vi "Facade.vi"(0 "Data In":T9, 2 "Display State In":T5, 3 "Container State":T8) -> (6 "Data Out":T9, 7 "Display State Out":T5, 8 "Action":T4)   [LabVIEW 2020, in "PXISlotGP.xctl"]
uses:
  PXISlotGP.xctl
  Data.ctl
  <vilib>/_xctls/Container State.ctl
  State.ctl
  PXISlot XControl/Connector Type.ctl
  AOAIRefs.ctl
  <vilib>/_xctls/Action.ctl
  <vilib>/_xctls/XControlSupport.lvlib
panel:
  in  "Tab panel":T1(tab) caption="SLOT X"
  in  "None":cluster{"String":string}
  in  "PXI-4461":T2 caption="Slot X"
  in  "BNC-2110":T3 caption="Slot X"
  in  "BNC-2090":T3 caption="Slot X"
types:
  T1 = enum32{"None", "PXI-4461", "BNC-2110", "BNC-2090"}
  T2 = cluster{"AI0":u16, "AI1":u16, "AO0":u16, "AO1":u16}
  T3 = cluster{"AI0":u16, "AI1":u16, "AI2":u16, "AI3":u16, "AI4":u16, "AI5":u16, "AI6":u16, "AI7":u16, "AO0":u16, "AO1":u16, "Trigger":string}
  T4 = typedef "XControlSupport.lvlib/Action.ctl" = cluster{"Data Changed?":bool, "State Changed?":bool, "Action Name":string}
  T5 = typedef "PXISlotGP.xctl/State.ctl" = cluster{"Connector Type":T6, "Hide unused":bool, "Trigger Visible":bool, "TabRef":refnum<vi>, "ConnRefs":refnum<vi>[], "PaneRef":refnum<vi>, "AOAIRefs":T7[], "TriggerRefs":refnum<vi>[], "check data":bool, "Name":string, "Events":cluster{"Type changed":refnum<user-event>}}
  T6 = typedef "Connector Type.ctl" = enum16{"None", "PXI-4461", "BNC-2110", "BNC-2090", "PXIe-4463", "PXIe-4464"}
  T7 = typedef "AOAIRefs.ctl" = cluster{"AORefs":refnum<vi>[], "AIRefs":refnum<vi>[]}
  T8 = typedef "XControlSupport.lvlib/Container State.ctl" = cluster{"Indicator?":bool, "Run Mode?":bool, " Refnum":refnum<vi>}
  T9 = typedef "PXISlotGP.xctl/Data.ctl" = cluster{"Outputs":string[], "Inputs":string[]}
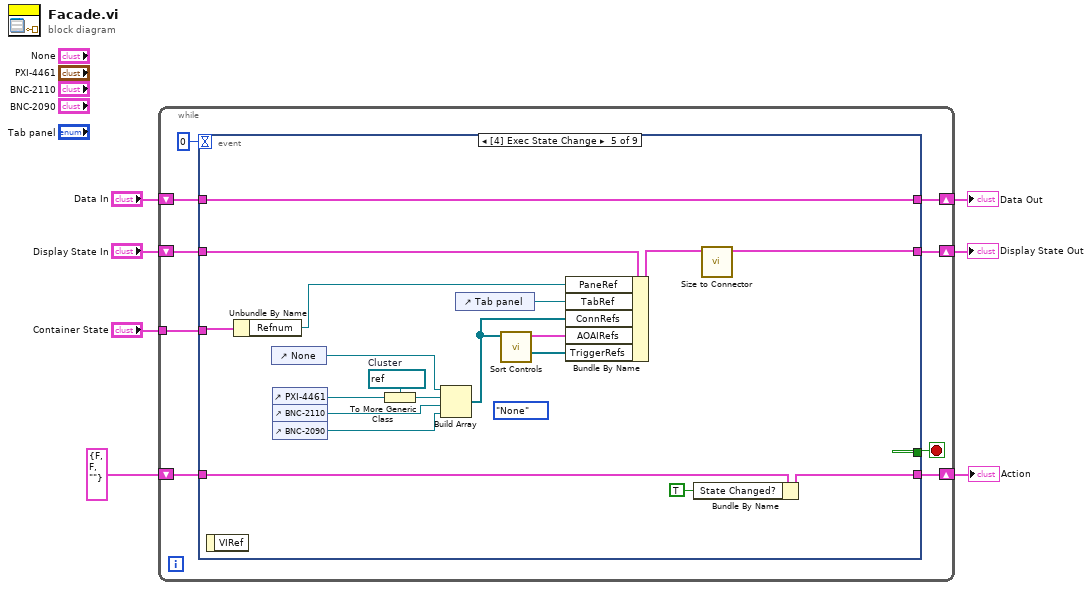
[diagram p0: block diagram]
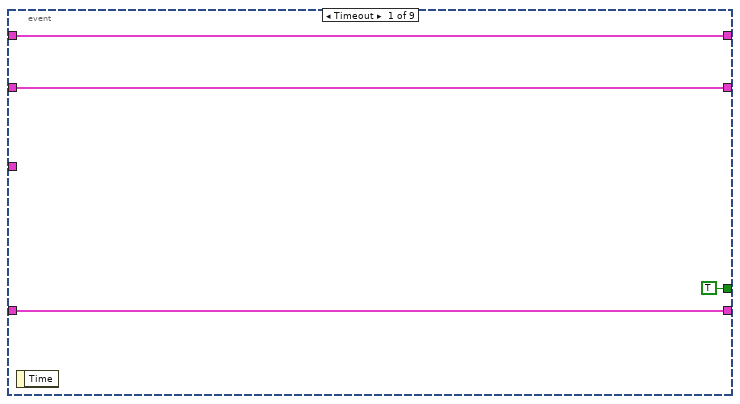
[diagram p2: hidden frame]
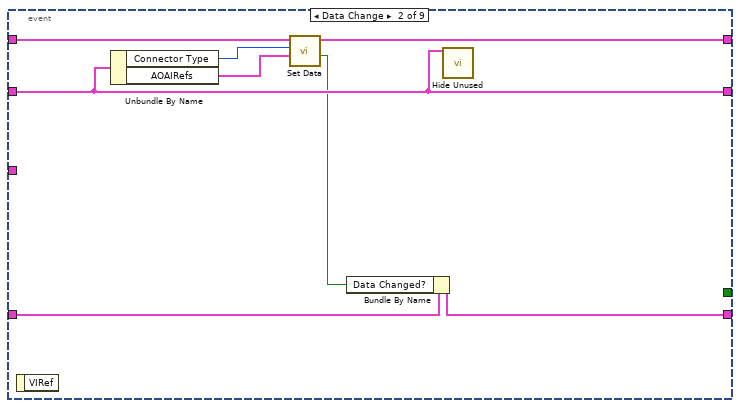
[diagram p3: hidden frame]
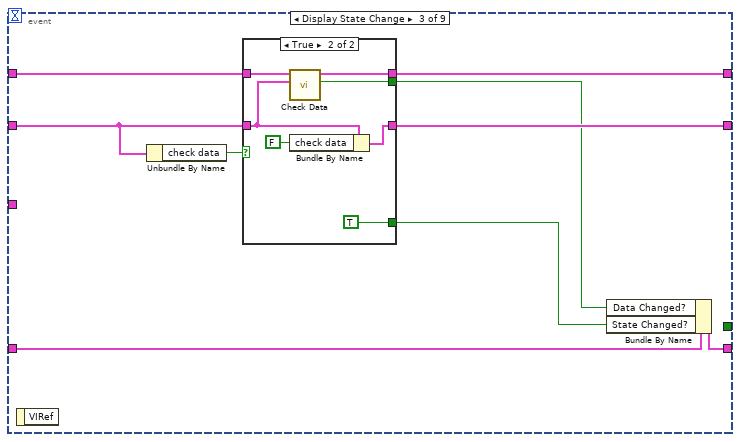
[diagram p4: hidden frame]
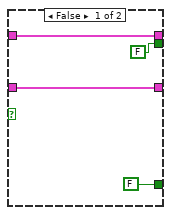
[diagram p5: hidden frame]
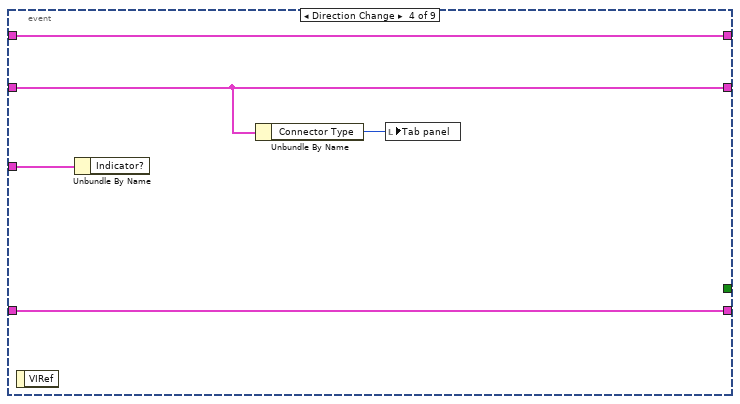
[diagram p6: hidden frame]
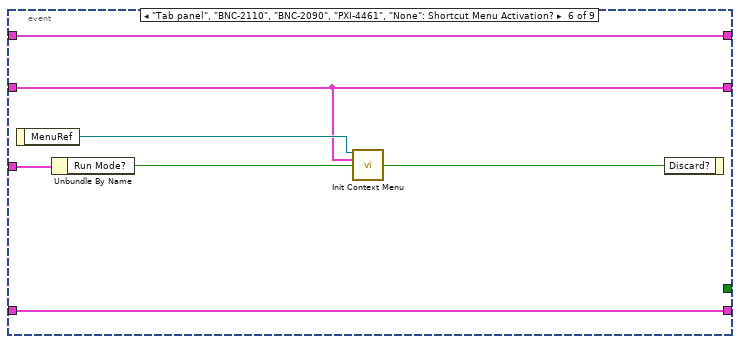
[diagram p7: hidden frame]
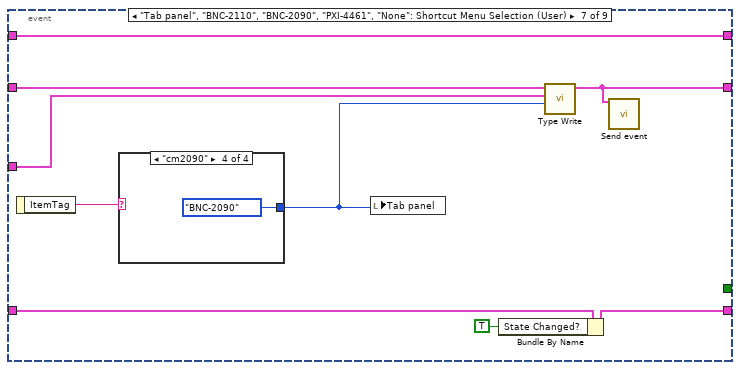
[diagram p8: hidden frame]
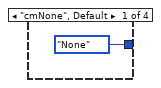
[diagram p9: hidden frame]
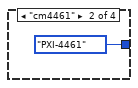
[diagram p10: hidden frame]
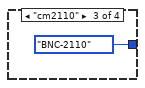
[diagram p11: hidden frame]
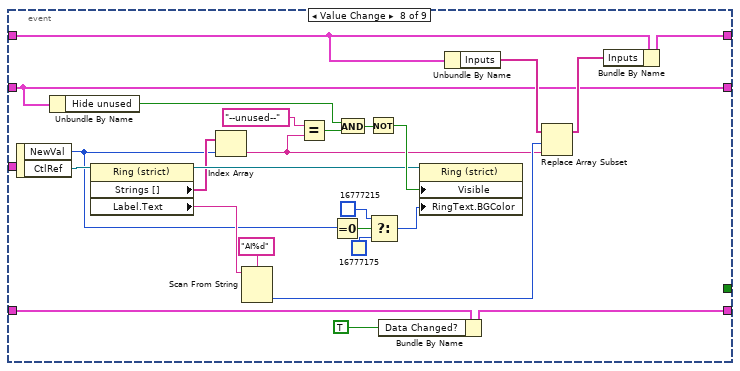
[diagram p12: hidden frame]
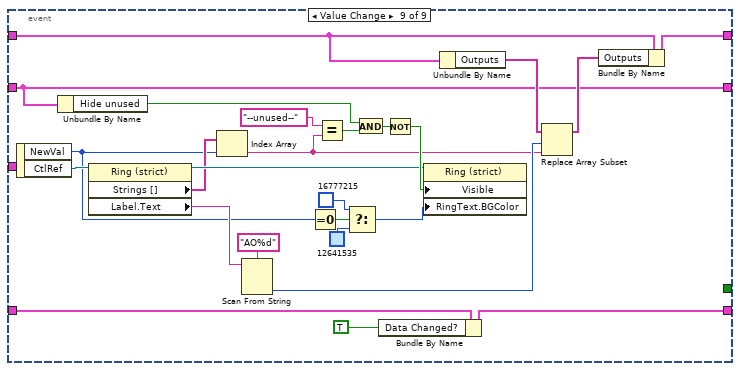
[diagram p13: hidden frame]
diagram:
  n1 = while {
    shift-right: [w15] -> w4
    shift-left: "Display State In" -> [w16]
    tunnel: "Container State" -> [w12]
    shift-right: [w10] -> w7
    shift-left: "Data In" -> [w11]
    shift-right: [w8] -> w2
    shift-left: T4 {"Data Changed?"=FALSE, "State Changed?"=FALSE, "Action Name"=""} ("Action") -> [w9]
    stop <- w14 stop-if-true
    n2 = event shown="[4] Exec State Change" {
      selector: _ -> [_ _ _ _ _ _ _ _ _]
      dyn-events: _ -> [_ _ _ _ _ _ _ _ _]
      timeout: 0 -> [_ _ _ _ _ _ _ _ _]
      tunnel: w16 -> [w18 w22 w36 w50 w72 w74 w83 w103 w129]
      tunnel: [w18 w22 w33 w50 w63 w74 w80 w103 w129] -> w15
      tunnel: [TRUE _ _ _ _ _ _ _ _] -> w14
      tunnel: w12 -> [_ _ _ w53 w66 w78 w82 _ _]
      tunnel: w11 -> [w17 w28 w35 w52 w71 w79 w88 w116 w141]
      tunnel: [w17 w27 w34 w52 w71 w79 w88 w114 w139] -> w10
      tunnel: [w19 w24 w32 w51 w68 w77 w85 w112 w137] -> w8
      tunnel: w9 -> [w19 w25 w37 w51 w70 w77 w87 w113 w138]
      event Timeout {
        n3 = event-data() -> ()  [unwired: 1 in, 1 out]
      }
      event Data Change {
        n4 = event-data() -> ()  [unwired: 1 in, 1 out]
        n5 = Unbundle By Name(w22) -> ("Connector Type"=w26:T6, "AOAIRefs"=w23:T7[])
        n6 = call "Set Data.vi"("AOAIRefs"=w23, "Connector Type"=w26, "Data"=w28) -> ("data changed"=w21:bool, "Data out"=w27:T9)  [unwired: 7 in]
        n7 = Bundle By Name(cluster=w25, "Data Changed?"=w21) -> (w24:T4)
        n8 = call "Hide Unused.vi"("Display State"=w22) -> ()  [unwired: 14 in, 1 out]
      }
      event Display State Change {
        n9 = event-data() -> ()  [unwired: 1 in, 1 out]
        n10 = Unbundle By Name(w36) -> ("check data"=w30:bool)
        n11 = case shown="True" w30 {
          tunnel: w36 -> [w40 w46]
          tunnel: w35 -> [w41 w48]
          tunnel: [w41 w47] -> w34
          tunnel: [w40 w45] -> w33
          tunnel: [FALSE TRUE] -> w31
          tunnel: [FALSE w42] -> w29
          frame False {
          }
          frame True {
            n12 = call "Check Data.vi"("Display State"=w46, "Data In"=w48) -> ("Changed"=w42:bool, "Data Out"=w47:T9)  [unwired: 8 in]
            n13 = Bundle By Name(cluster=w46, "check data"=FALSE) -> (w45:T5)
          }
        }
        n14 = Bundle By Name(cluster=w37, "Data Changed?"=w29, "State Changed?"=w31) -> (w32:T4)
      }
      event Direction Change {
        n15 = event-data() -> ()  [unwired: 1 in, 1 out]
        n16 = Unbundle By Name(w53) -> ()  [unwired: 1 out]
        n17 = Unbundle By Name(w50) -> ("Connector Type"=w49:T6)
        n18 = local write "Tab panel"(w49) -> ()
      }
      event Exec State Change {
        (unwired) Connector_Type."None" ("Connector Type")
        w60 = refnum<vi> refnum  # Cluster
        n19 = event-data() -> ()  [unwired: 1 in, 1 out]
        n20 = Unbundle By Name(w66) -> ("Refnum"=w65:refnum<vi>)
        n21 = control-ref of="None"() -> (w54:refnum<vi>)
        n22 = control-ref of="PXI-4461"() -> (w56:refnum<vi>)
        n23 = control-ref of="BNC-2110"() -> (w57:refnum<vi>)
        n24 = control-ref of="BNC-2090"() -> (w58:refnum<vi>)
        n25 = To More Generic Class(target class=w60, reference=w56) -> (generic class reference=w59:refnum<vi>)
        n26 = Build Array(w54, w59, w57, w58) -> (w55:refnum<vi>[])
        n27 = control-ref of="Tab panel"() -> (w69:refnum<vi>)
        n28 = call "Sort Controls.vi"("ConnRefs"=w55) -> ("TriggerRefs"=w61:refnum<vi>[], "AOAIRefs"=w62:T7[])  [unwired: 9 in]
        n29 = Bundle By Name(cluster=w72, "PaneRef"=w65, "TabRef"=w69, "ConnRefs"=w55, "AOAIRefs"=w62, "TriggerRefs"=w61) -> (w64:T5)
        n30 = Bundle By Name(cluster=w70, "State Changed?"=TRUE) -> (w68:T4)
        n31 = call "Size to Connector.vi"("Display State In in"=w64) -> ("Display State In out"=w63:T5)  [unwired: 9 in, 1 out]
      }
      event "Tab panel", "BNC-2110", "BNC-2090", "PXI-4461", "None": Shortcut Menu Activation? {
        n32 = event-data() -> ("MenuRef"=w75:refnum<k9>)  [unwired: 1 in]
        n33 = Unbundle By Name(w78) -> ("Run Mode?"=w76:bool)
        n34 = call "Init Context Menu.vi"("Menu in"=w75, "Display State In"=w74, "Run Mode?"=w76) -> ("Discard"=w73:bool)  [unwired: 11 in, 1 out]
        n35 = event-data("Discard?"=w73) -> ()  [unwired: 1 in, 1 out]
      }
      event "Tab panel", "BNC-2110", "BNC-2090", "PXI-4461", "None": Shortcut Menu Selection (User) {
        n36 = event-data() -> ("ItemTag"=w86:string)  [unwired: 1 in]
        n37 = case shown="\"cm2090\"" w86 {
          tunnel: [T1."None" ("PXISlot Control") T1."PXI-4461" ("PXISlot Control") T1."BNC-2110" ("PXISlot Control") T1."BNC-2090" ("PXISlot Control")] -> w81
          frame "cmNone", Default {
          }
          frame "cm4461" {
          }
          frame "cm2110" {
          }
          frame "cm2090" {
          }
        }
        n38 = local write "Tab panel"(w81) -> ()
        n39 = Bundle By Name(cluster=w87, "State Changed?"=TRUE) -> (w85:T4)
        n40 = call "Type Write.vi"("Value"=w81, "Container State"=w82, "Display State In"=w83) -> ("Display State Out"=w80:T5)  [unwired: 3 in, 1 out]
        n41 = call "Send event.vi"("State"=w80) -> ()  [unwired: 14 in, 1 out]
      }
      event "BNC-2110.AI0", "BNC-2110.AI1", "BNC-2110.AI2", "BNC-2110.AI3", "BNC-2110.AI4", "BNC-2110.AI5", "BNC-2110.AI6", "BNC-2110.AI7", "PXI-4461.AI0", "PXI-4461.AI1", "BNC-2090.AI0", "BNC-2090.AI1", "BNC-2090.AI2", "BNC-2090.AI3", "BNC-2090.AI4", "BNC-2090.AI5", "BNC-2090.AI6", "BNC-2090.AI7": Value Change {
        n42 = event-data() -> ("NewVal"=w93:u16, "CtlRef"=w107:refnum<vi>)  [unwired: 1 in]
        n43 = Unbundle By Name(w103) -> ("Hide unused"=w108:bool)
        n44 = property class="Ring (strict)"(reference=w107) -> (reference out=w99:refnum<vi>, "Strings []"=w98:string[], "Label.Text"=w100:string)  [unwired: 1 in, 1 out]
        n45 = Index Array(array=w98, index=w93) -> (element=w102:string)
        n46 = Scan From String(format string="AI%d", input string=w100) -> (output 1=w110:i32)  [unwired: 3 in, 3 out]
        n47 = Equal?(x="--unused--", y=w102) -> (x = y?=w109:bool)
        n48 = Equal To 0?(x=w93) -> (x = 0?=w97:bool)
        n49 = And(x=w108, y=w109) -> (x .and. y?=w106:bool)
        n50 = Not(x=w106) -> (.not. x?=w105:bool)
        n51 = Select(t=u32 16777215, s=w97, f=u32 16777175) -> (s? t:f=w94:u32)
        n52 = Bundle By Name(cluster=w113, "Data Changed?"=TRUE) -> (w112:T4)
        n53 = property class="Ring (strict)"(reference=w99, "Visible"=w105, "RingText.BGColor"=w94) -> ()  [unwired: 1 in, 2 out]
        n54 = Unbundle By Name(w116) -> ("Inputs"=w117:string[])
        n55 = Replace Array Subset(array=w117, new element=w102, index=w110) -> (w115:string[])
        n56 = Bundle By Name(cluster=w116, "Inputs"=w115) -> (w114:T9)
      }
      event "BNC-2110.AO0", "BNC-2110.AO1", "PXI-4461.AO0", "PXI-4461.AO1", "BNC-2090.AO0", "BNC-2090.AO1": Value Change {
        n57 = event-data() -> ("NewVal"=w119:u16, "CtlRef"=w126:refnum<vi>)  [unwired: 1 in]
        n58 = Unbundle By Name(w129) -> ("Hide unused"=w133:bool)
        n59 = property class="Ring (strict)"(reference=w126) -> (reference out=w125:refnum<vi>, "Strings []"=w123:string[], "Label.Text"=w124:string)  [unwired: 1 in, 1 out]
        n60 = Index Array(array=w123, index=w119) -> (element=w128:string)
        n61 = Scan From String(format string="AO%d", input string=w124) -> (output 1=w135:i32)  [unwired: 3 in, 3 out]
        n62 = Equal To 0?(x=w119) -> (x = 0?=w122:bool)
        n63 = Equal?(x="--unused--", y=w128) -> (x = y?=w134:bool)
        n64 = Select(t=u32 16777215, s=w122, f=u32 12641535) -> (s? t:f=w118:u32)
        n65 = And(x=w133, y=w134) -> (x .and. y?=w132:bool)
        n66 = Bundle By Name(cluster=w138, "Data Changed?"=TRUE) -> (w137:T4)
        n67 = Not(x=w132) -> (.not. x?=w131:bool)
        n68 = property class="Ring (strict)"(reference=w125, "Visible"=w131, "RingText.BGColor"=w118) -> ()  [unwired: 1 in, 2 out]
        n69 = Unbundle By Name(w141) -> ("Outputs"=w142:string[])
        n70 = Replace Array Subset(array=w142, new element=w128, index=w135) -> (w140:string[])
        n71 = Bundle By Name(cluster=w141, "Outputs"=w140) -> (w139:T9)
      }
    }
  }
  "Display State Out" <- w4
  "Data Out" <- w7
  "Action" <- w2
